vi "rateFilter_FPGA.vi"(7 "maxDiff":fxp<+/-,16,9>, 11 "Angle in":fxp<+/-,16,9>) -> (3 "Angle out":fxp<+/-,16,9>)   [LabVIEW 2016]
uses:
  <vilib>/rvi/FXPMathLib/FxpSub/XNode/nifxpmath_Sub.xnode
  <vilib>/rvi/FXPMathLib/FxpMul/XNode/nifxpmath_Multiplier.xnode
  <vilib>/rvi/FXPMathLib/FxpAdd/XNode/nifxpmath_Add.xnode
  <vilib>/rvi/FXPMathLib/sim/FxpSim.dll
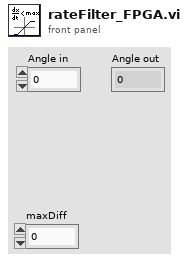
[diagram p1: front panel]
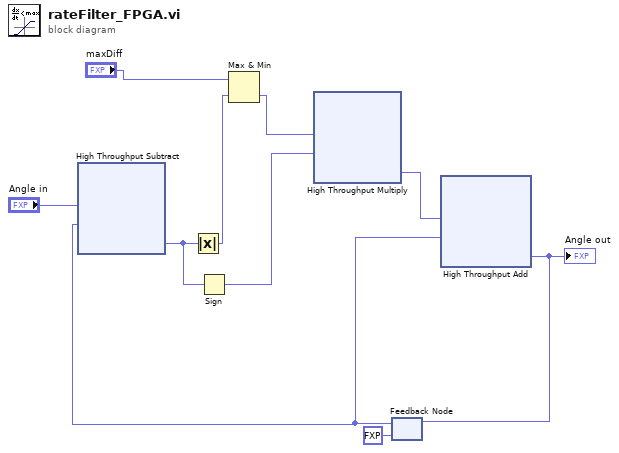
[diagram p0: block diagram]
diagram:
  n1 = feedback #1(fxp<+/-,16,9> 0.0) -> (w1:fxp<+/-,16,9>)
  n2 = xnode "High Throughput Subtract"("x"="Angle in", "y"=w1) -> ("x-y"=w6:fxp<+/-,16,9>)
  n3 = Absolute Value(x=w6) -> (abs(x)=w7:fxp<+,16,9>)
  n4 = Sign(1:w6) -> (0:w4:fxp<+/-,2,2>)
  n5 = Max & Min(x="maxDiff", y=w7) -> (min(x,y)=w5:fxp<+/-,17,10>)  [unwired: 1 out]
  n6 = xnode "High Throughput Multiply"("x"=w5, "y"=w4) -> ("x*y"=w3:fxp<+/-,16,9>)
  n7 = xnode "High Throughput Add"("x"=w3, "y"=w1) -> ("x+y"=w2:fxp<+/-,16,9>)
  "Angle out" <- w2
  n8 = feedback-in #1(w2) -> ()
